vi "rio.vi"() -> ()   [LabVIEW 2012]
uses:
  <vilib>/rvi/interface/nirviOpenFPGA/nirviOpenFPGA.xnode
  <vilib>/rvi/interface/nirviMethod/nirviMethod.xnode
  <vilib>/rvi/interface/nirviReadWriteControl/nirviReadWriteControl.xnode
  <vilib>/addons/Fuzzy Logic/NI_Fuzzy_Logic_API.lvlib
  RIOGlobal.vi
  <vilib>/addons/Fuzzy Logic/TypeDefs/FL Interpolating polynomials.ctl
  <vilib>/addons/Fuzzy Logic/TypeDefs/FL Defuzzification.ctl
  <vilib>/addons/Fuzzy Logic/TypeDefs/FL Consequent Implication.ctl
  <vilib>/addons/Fuzzy Logic/TypeDefs/FL Modifier.ctl
  <vilib>/addons/Fuzzy Logic/TypeDefs/FL Consequent.ctl
  <vilib>/addons/Fuzzy Logic/TypeDefs/FL Antecedent Connective.ctl
  <vilib>/addons/Fuzzy Logic/TypeDefs/FL Antecedent.ctl
  <vilib>/addons/Fuzzy Logic/TypeDefs/FL Rule.ctl
  <vilib>/addons/Fuzzy Logic/TypeDefs/FL Membership Function Shape.ctl
  <vilib>/addons/Fuzzy Logic/TypeDefs/FL Membership Function.ctl
  <vilib>/addons/Fuzzy Logic/TypeDefs/FL Variable.ctl
  <vilib>/addons/Fuzzy Logic/TypeDefs/FL System.ctl
  <vilib>/FPGAPlugInAG/Dynamic/niLvFpga_Reset_Dynamic.vi
  <vilib>/rvi/interface/Simulation/niFpgaSimulationCallBeginRW.vi
  <vilib>/rvi/errors/niLvFpgaAdjustHostInterfaceError.vi
  <vilib>/FPGAPlugInAG/Dynamic/niLvFpga_Run_Dynamic.vi
  <vilib>/Utility/error.llb/Error Cluster From Error Code.vi
  NiFpgaLv.dll
  <vilib>/FPGAPlugInAG/Dynamic/niLvFpga_ReadFifo_Dynamic.vi
  <vilib>/rvi/errors/niLvFpgaMergeErrorWithErrorCode.vi
  logcode/G_read.vi
  <vilib>/FPGAPlugInAG/Dynamic/niLvFpga_StartFifo_Dynamic.vi
  <vilib>/addons/Fuzzy Logic/FL Fuzzy Controller (MISO).vi
  FPGA Bitfiles/autonomous_FPGATarget_autofpga8_egKHF51X6I0.lvbitx
  autocarnav4/soul/fpga/autofpga8.vi
  <vilib>/FPGAPlugInAG/cRIO-9114/niLvFpga_Open_cRIO-9114.vi
  <vilib>/rvi/interface/common/dynamic/niFpgaDynamicAddResources.vi
panel:
  out "get position":bool
  out "get heading":bool
  out "inbound?":bool
  in  "pos_error_bound gain":dbl=500.0
  out "LCC":dbl[](array[numeric]) format="%#_19f"
  out "tempheading":dbl
  in  "Buzz":bool=TRUE
  out "Steering_masual":dbl
  out "Steering_Des":dbl
  out "VS_Des":dbl
  out "Auto":bool
  out "Run":bool
  out "E - STOP":bool
  out "FPGA error out":errorcluster
  out "FPGA VI Reference Out":refnum<k20>
  out "bias":dbl
  in  "pos init manual":bool=TRUE
  out "hor.std.":dbl
  out "h_gps":dbl
  out "pos linit":bool
  out "dt":dbl
  out "ecef ref":dbl[](array[numeric])
  out "heading linit":bool
  out "time":i16
  out "output":T1
  in  "file write":bool
  out "refnum out":refnum<file>
  out "error out":errorcluster
  in  "position weight":dbl=0.1
  in  "heading weight":dbl=0.1
  out "rt":dbl
  out "steer_MDPS":dbl
  out "B Push percent x10":dbl
  in  "Slide":dbl(slide) scale=0.0..100.0
  in  "brake filter":dbl=1.0
  in  "Knob steer":dbl(knob)=122.29647676637626 scale=-550.0..550.0
  in  "knob steer":bool
  in  "auto brake":bool=TRUE
  in  "auto speed":bool=TRUE
  out "VS_TCU":dbl
  in  "auto steer":bool=TRUE
  out "Throttle Enable":bool=TRUE
  in  "VS_maual":dbl=33.0
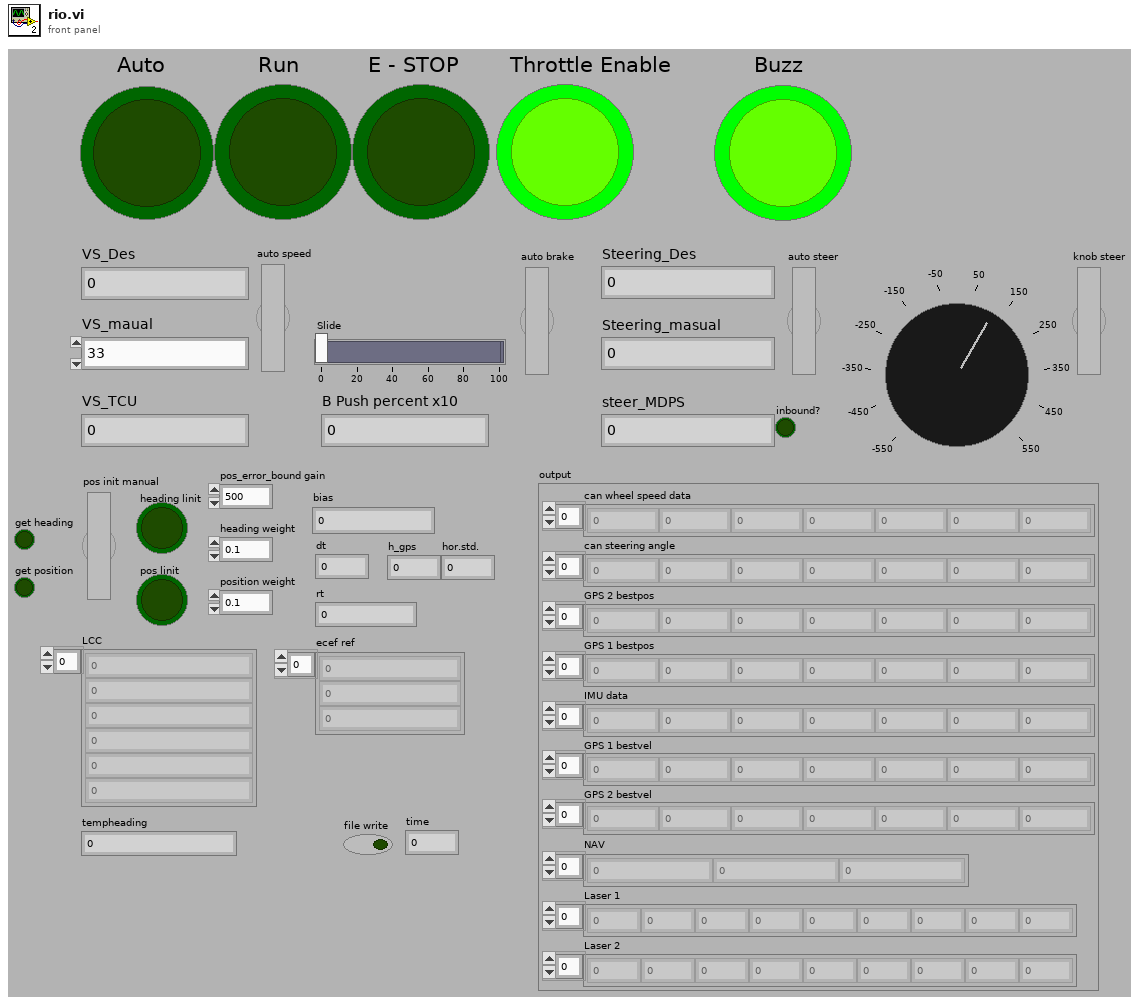
[diagram p1: front panel]
types:
  T1 = cluster{"can wheel speed data":u8[], "can steering angle":i32[], "GPS 2 bestpos":u8[], "GPS 1 bestpos":u8[], "IMU data":i16[], "GPS 1 bestvel":u8[], "GPS 2 bestvel":u8[], "NAV":dbl[], "Laser 1":u16[], "Laser 2":u16[]}
  T2 = typedef "NI_Fuzzy_Logic_API.lvlib/FL System.ctl" = cluster{"input variables":T3[], "output variables":T3[], "rules":T6[], "defuzzification method":T12, "description":string, "user MF interpolating polynomials":T13[]}
  T3 = typedef "NI_Fuzzy_Logic_API.lvlib/FL Variable.ctl" = cluster{"name":string, "range":dbl[], "MFs":T4[]}
  T4 = typedef "NI_Fuzzy_Logic_API.lvlib/FL Membership Function.ctl" = cluster{"name":string, "shape":T5, "points":dbl[], "color":u32, "user-defined shape index":i32}
  T5 = typedef "NI_Fuzzy_Logic_API.lvlib/FL Membership Function Shape.ctl" = u16
  T6 = typedef "NI_Fuzzy_Logic_API.lvlib/FL Rule.ctl" = cluster{"antecedents":T7[], "antecedent connective":T9, "consequents":T10[], "consequent implication":T11, "degree of support":dbl}
  T7 = typedef "NI_Fuzzy_Logic_API.lvlib/FL Antecedent.ctl" = cluster{"Var Index":i32, "MF Index":i32, "Cond":T8}
  T8 = typedef "NI_Fuzzy_Logic_API.lvlib/FL Modifier.ctl" = u16
  T9 = typedef "NI_Fuzzy_Logic_API.lvlib/FL Antecedent Connective.ctl" = u16
  T10 = typedef "NI_Fuzzy_Logic_API.lvlib/FL Consequent.ctl" = cluster{"Var Index":i32, "MF Index":i32, "Cond":T8}
  T11 = typedef "NI_Fuzzy_Logic_API.lvlib/FL Consequent Implication.ctl" = u16
  T12 = typedef "NI_Fuzzy_Logic_API.lvlib/FL Defuzzification.ctl" = u16
  T13 = typedef "NI_Fuzzy_Logic_API.lvlib/FL Interpolating polynomials.ctl" = cluster{"X":dbl[], "Y":dbl[], "Y(x) coeff":dbl[][], "X(y) coeff":dbl[][], "Area(y) coeff":dbl[][], "coa_x(y) coeff":dbl[][]}
  T14 = enum16{"open", "replace", "create", "open or create", "replace or create", "replace or create with confirmation"}
  T15 = cluster{"counter[ms]":u16, "rate x[rad/sec]":i16, "rate y[rad/sec]":i16, "rate z[rad/sec]":i16, "accel x[m/s^2]":i16, "accel y[m/s^2]":i16, "accel z[m/s^2]":i16}
  T16 = cluster{"counter[ms]":i16, "rate x[rad/sec]":i16, "rate y[rad/sec]":i16, "rate z[rad/sec]":i16, "accel x[m/s^2]":i16, "accel y[m/s^2]":i16, "accel z[m/s^2]":i16}
  T17 = cluster{"sol stat":u32, "vel type":u32, "latency":sgl, "age":sgl, "hor spd":dbl, "trk gnd":dbl, "vert spd":dbl, "reserved":sgl, "CRC":u32}
  T18 = cluster{"Sync_AA":u8, "Sync_44":u8, "Sync_12":u8, "Header Lgth":u8, "Message ID":u16, "Message Type":u8, "Port Address":u8, "Message Length":u16, "Sequence":u16, "Idle Time":u8, "Time Status":u8, "Week":u16, "ms":u32, "Receiver Status":u32, "Reserved":u16, "Receiver S/W Version":u16}
  T19 = cluster{"sol stat":u32, "pos type":u32, "lat":dbl, "lon":dbl, "hgt":dbl, "undulation":sgl, "dataum id":u32, "lat dev":sgl, "lon dev":sgl, "hgt dev":sgl, "stn id":u32, "diff_age":sgl, "sol_age":sgl, "#SVs":u8, "#solnSVs":u8, "#solnL1SVs":u8, "#solnMultiSVs":u8, "Reserved":u8, "ext sol stat":u8, "Reserved 2":u8, "sig mask":u8, "CRC":u32}
  T20 = cluster{"can wheel speed data":u8[], "can steering angle":i32[], "GPS 2 bestpos":u8[], "GPS 1 bestpos":u8[], "IMU data":i16[], "GPS 1 bestvel":u8[], "GPS 2 bestvel":u8[]}
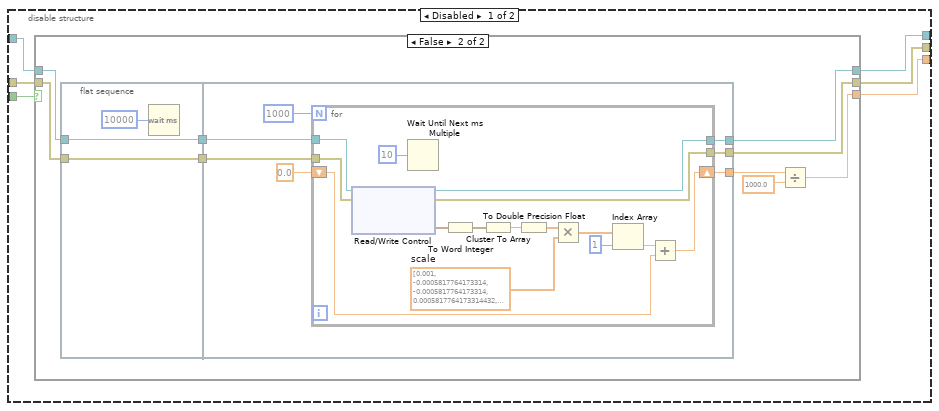
[diagram p2: hidden frame]
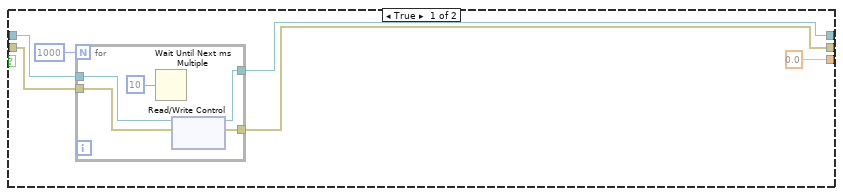
[diagram p3: hidden frame]
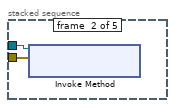
[diagram p4: hidden frame]
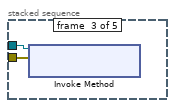
[diagram p5: hidden frame]
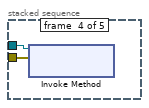
[diagram p6: hidden frame]
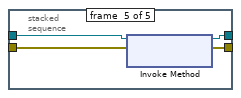
[diagram p7: hidden frame]
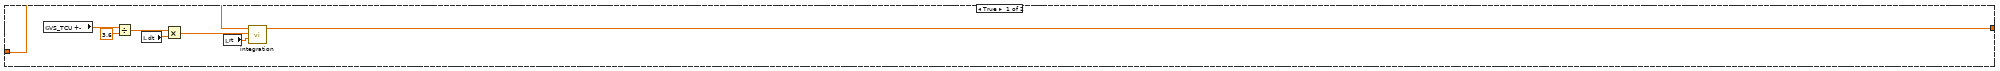
[diagram p12: hidden frame]
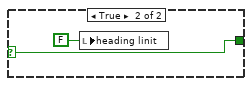
[diagram p13: hidden frame]
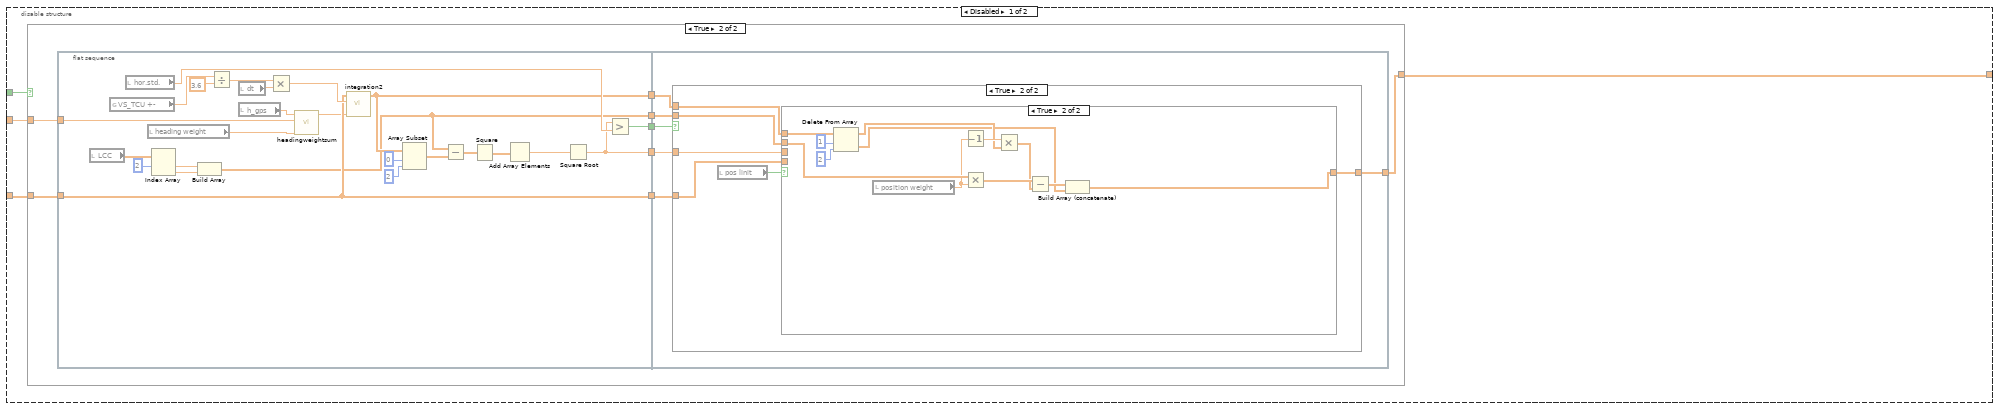
[diagram p14: hidden frame]
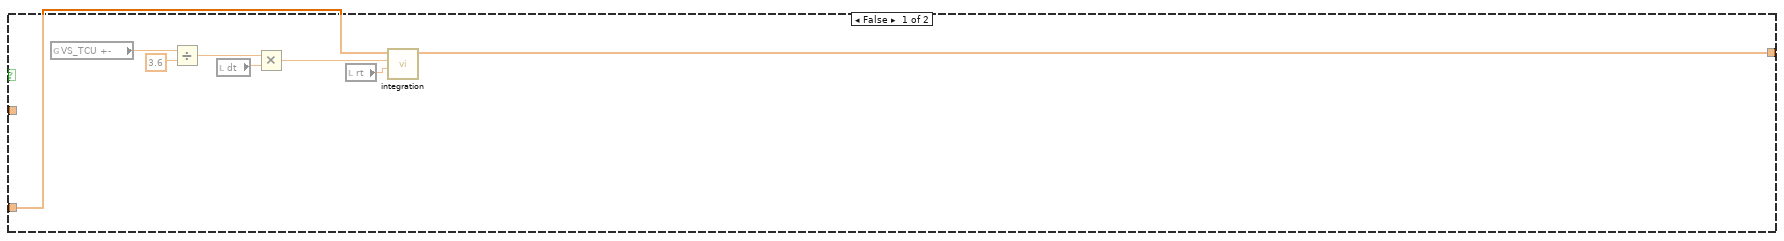
[diagram p15: hidden frame]
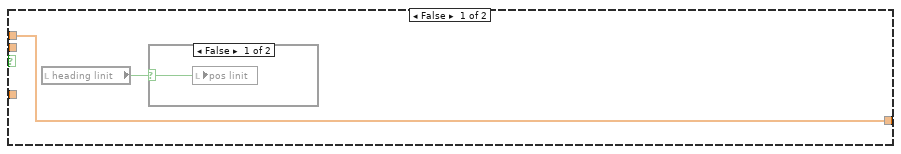
[diagram p16: hidden frame]
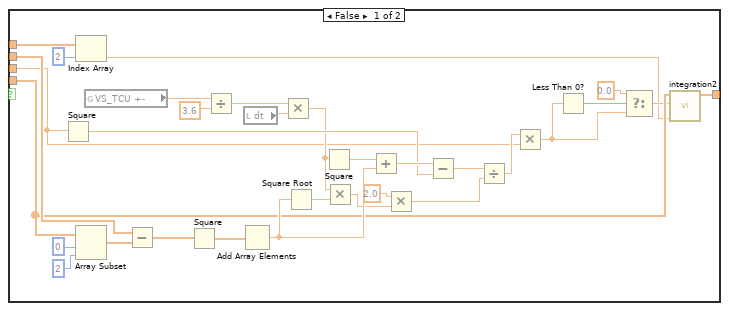
[diagram p18: hidden frame]
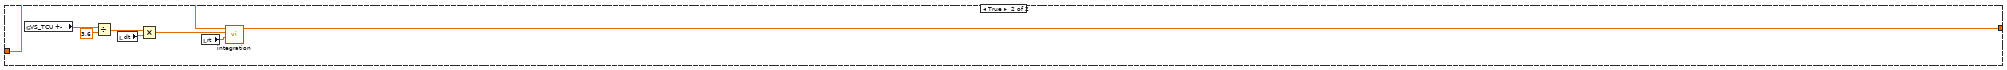
[diagram p19: hidden frame]
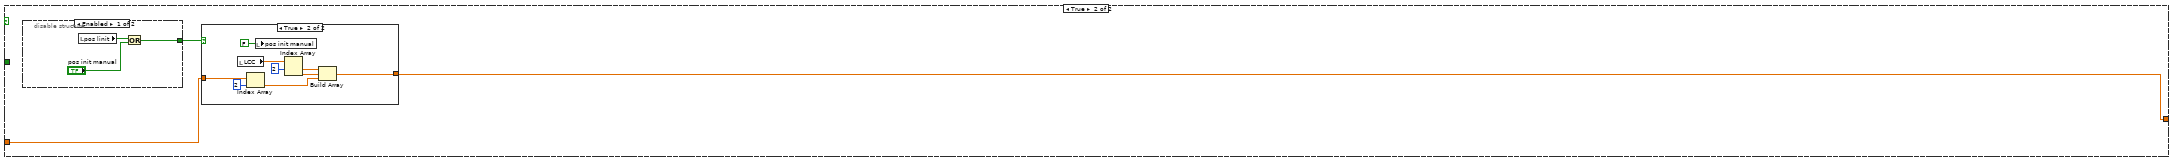
[diagram p20: hidden frame]
diagram:
  n1 = flat-sequence {
    tunnel: [T2 {"input variables"=[{"name"="Vdes-Vcar", "range"=[-100.0, 100.0, -150.0, 150.0], "MFs"=[{"name"="TF", "shape"=0, "points"=[-150.0, -10.0, -5.0], "color"=0, "user-defined shape index"=0}, {"name"="FR", "shape"=0, "points"=[-10.0, -5.0, 0.0], "color"=12369084, "user-defined shape index"=0}, {"name"="TR", "shape"=0, "points"=[-5.0, 0.0, 5.0], "color"=16711680, "user-defined shape index"=0}, {"name"="SR", "shape"=0, "points"=[0.0, 5.0, 10.0], "color"=6618880, "user-defined shape index"=0}, {"name"="TS", "shape"=0, "points"=[5.0, 10.0, 150.0], "color"=1985280, "user-defined shape index"=0}]}, {"name"="Vdes", "range"=[0.0, 10.0, -0.5, 100.0], "MFs"=[{"name"="ST", "shape"=0, "points"=[-0.5, 0.0, 0.5], "color"=16860, "user-defined shape index"=0}, {"name"="CR", "shape"=0, "points"=[0.0, 3.0, 6.0], "color"=16776704, "user-defined shape index"=0}, {"name"="DR", "shape"=0, "points"=[0.5, 10.0, 100.0], "color"=7171459, "user-defined shape index"=0}]}], "output variables"=[{"name"="BrakeAngle", "range"=[-5.0, 90.0, -5.0, 120.0], "MFs"=[{"name"="NB", "shape"=0, "points"=[-5.0, 0.0, 4.0], "color"=11121611, "user-defined shape index"=0}, {"name"="LB", "shape"=0, "points"=[0.0, 10.0, 20.0], "color"=11776947, "user-defined shape index"=0}, {"name"="MB", "shape"=0, "points"=[5.0, 35.0, 65.0], "color"=3381759, "user-defined shape index"=0}, {"name"="FB", "shape"=0, "points"=[20.0, 70.0, 120.0], "color"=32639, "user-defined shape index"=0}]}], "rules"=[{"antecedents"=[{"Var Index"=0, "MF Index"=0, "Cond"=0}, {"Var Index"=1, "MF Index"=0, "Cond"=0}], "antecedent connective"=0, "consequents"=[{"Var Index"=0, "MF Index"=3, "Cond"=0}], "consequent implication"=0, "degree of support"=1.0}, {"antecedents"=[{"Var Index"=0, "MF Index"=1, "Cond"=0}, {"Var Index"=1, "MF Index"=0, "Cond"=0}], "antecedent connective"=0, "consequents"=[{"Var Index"=0, "MF Index"=3, "Cond"=0}], "consequent implication"=0, "degree of support"=1.0}, {"antecedents"=[{"Var Index"=0, "MF Index"=2, "Cond"=0}, {"Var Index"=1, "MF Index"=0, "Cond"=0}], "antecedent connective"=0, "consequents"=[{"Var Index"=0, "MF Index"=2, "Cond"=0}], "consequent implication"=0, "degree of support"=1.0}, {"antecedents"=[{"Var Index"=0, "MF Index"=3, "Cond"=0}, {"Var Index"=1, "MF Index"=0, "Cond"=0}], "antecedent connective"=0, "consequents"=[{"Var Index"=0, "MF Index"=3, "Cond"=0}], "consequent implication"=0, "degree of support"=1.0}, {"antecedents"=[{"Var Index"=0, "MF Index"=4, "Cond"=0}, {"Var Index"=1, "MF Index"=0, "Cond"=0}], "antecedent connective"=0, "consequents"=[{"Var Index"=0, "MF Index"=3, "Cond"=0}], "consequent implication"=0, "degree of support"=1.0}, {"antecedents"=[{"Var Index"=0, "MF Index"=0, "Cond"=0}, {"Var Index"=1, "MF Index"=1, "Cond"=0}], "antecedent connective"=0, "consequents"=[{"Var Index"=0, "MF Index"=3, "Cond"=0}], "consequent implication"=0, "degree of support"=1.0}, {"antecedents"=[{"Var Index"=0, "MF Index"=1, "Cond"=0}, {"Var Index"=1, "MF Index"=1, "Cond"=0}], "antecedent connective"=0, "consequents"=[{"Var Index"=0, "MF Index"=2, "Cond"=0}], "consequent implication"=0, "degree of support"=1.0}, {"antecedents"=[{"Var Index"=0, "MF Index"=2, "Cond"=0}, {"Var Index"=1, "MF Index"=1, "Cond"=0}], "antecedent connective"=0, "consequents"=[{"Var Index"=0, "MF Index"=1, "Cond"=0}], "consequent implication"=0, "degree of support"=1.0}, {"antecedents"=[{"Var Index"=0, "MF Index"=3, "Cond"=0}, {"Var Index"=1, "MF Index"=1, "Cond"=0}], "antecedent connective"=0, "consequents"=[{"Var Index"=0, "MF Index"=0, "Cond"=0}], "consequent implication"=0, "degree of support"=1.0}, {"antecedents"=[{"Var Index"=0, "MF Index"=4, "Cond"=0}, {"Var Index"=1, "MF Index"=1, "Cond"=0}], "antecedent connective"=0, "consequents"=[{"Var Index"=0, "MF Index"=0, "Cond"=0}], "consequent implication"=0, "degree of support"=1.0}, {"antecedents"=[{"Var Index"=0, "MF Index"=0, "Cond"=0}, {"Var Index"=1, "MF Index"=2, "Cond"=0}], "antecedent connective"=0, "consequents"=[{"Var Index"=0, "MF Index"=3, "Cond"=0}], "consequent implication"=0, "degree of support"=1.0}, {"antecedents"=[{"Var Index"=0, "MF Index"=1, "Cond"=0}, {"Var Index"=1, "MF Index"=2, "Cond"=0}], "antecedent connective"=0, "consequents"=[{"Var Index"=0, "MF Index"=2, "Cond"=0}], "consequent implication"=0, "degree of support"=1.0}, {"antecedents"=[{"Var Index"=0, "MF Index"=2, "Cond"=0}, {"Var Index"=1, "MF Index"=2, "Cond"=0}], "antecedent connective"=0, "consequents"=[{"Var Index"=0, "MF Index"=0, "Cond"=0}], "consequent implication"=0, "degree of support"=1.0}, {"antecedents"=[{"Var Index"=0, "MF Index"=3, "Cond"=0}, {"Var Index"=1, "MF Index"=2, "Cond"=0}], "antecedent connective"=0, "consequents"=[{"Var Index"=0, "MF Index"=0, "Cond"=0}], "consequent implication"=0, "degree of support"=1.0}, {"antecedents"=[{"Var Index"=0, "MF Index"=4, "Cond"=0}, {"Var Index"=1, "MF Index"=2, "Cond"=0}], "antecedent connective"=0, "consequents"=[{"Var Index"=0, "MF Index"=0, "Cond"=0}], "consequent implication"=0, "degree of support"=1.0}], "defuzzification method"=0, "description"="", "user MF interpolating polynomials"=[]} ("fuzzy system out")] -> w1
    tunnel: w1 -> [w113]
    frame #0 {
      n2 = flat-sequence {
        frame #0 {
          w110 = TRUE ("auto steer")
          n3 = call "getecefdcmref.vi"("map"=2) -> ("XYZ"=→"ecef ref":dbl[])  [unwired: 10 in, 4 out]
          n4 = local write "Knob steer"(0.0 ("Knob steer")) -> ()
          n5 = local write "knob steer"(FALSE ("knob steer")) -> ()
          n6 = shared-variable "cRIO-9024\\sharedvari.lvlib\\parked"(FALSE ("parked")) -> ()  [unwired: 1 in, 1 out]
          n7 = local write "VS_maual"(32.0 ("VS_Desire")) -> ()
          n8 = global write "RIOGlobal.vi" "amp_ini"(2.5 ("amp_ini")) -> ()
          n9 = local write "Buzz"(w110) -> ()
          n10 = local write "auto steer"(w110) -> ()
          n11 = local write "auto speed"(w110) -> ()
          n12 = local write "auto brake"(w110) -> ()
          "heading linit" <- TRUE
          "pos linit" <- TRUE
        }
      }
      n13 = flat-sequence {
        frame #0 {
          n14 = xnode "Open FPGA VI Reference"() -> ("FPGA VI Reference Out"=w22:refnum<k20>, "error out"=w21:errorcluster)  [unwired: 2 in]
          n15 = xnode "Invoke Method"("FPGA VI Reference In"=w22, "error in"=w21) -> ("FPGA VI Reference Out"=w20:refnum<k20>, "error out"=w19:errorcluster)
          n16 = xnode "Read/Write Control"("FPGA VI Reference In"=w20, "error in"=w19, "read can"=TRUE, "16k"=FALSE) -> ("FPGA VI Reference Out"=w18:refnum<k20>, "error out"=w17:errorcluster)
          n17 = xnode "Invoke Method"("FPGA VI Reference In"=w18, "error in"=w17) -> ("FPGA VI Reference Out"=w15:refnum<k20>, "error out"=w14:errorcluster)  [unwired: 1 in]
          n18 = while {
            tunnel: w15 -> [w95]
            tunnel: w14 -> [w94]
            tunnel: [w93] -> w9
            tunnel: [w90] -> w10
            stop <- w91 stop-if-true
            n19 = xnode "Read/Write Control"("FPGA VI Reference In"=w95, "error in"=w94) -> ("FPGA VI Reference Out"=w90:refnum<k20>, "error out"=w93:errorcluster, "amp"=w92:fxp<+/-,16,5>)
            n20 = Not Equal To 0?(x=w92) -> (x != 0?=w91:bool)
          }
          n21 = stacked-sequence {
            tunnel: w10 -> [w79 w81 w83 w85 w89]
            tunnel: w9 -> [w78 w80 w82 w84 w88]
            tunnel: [_ _ _ _ w87] -> w7
            tunnel: [_ _ _ _ w86] -> w6
            frame #0 {
              n22 = xnode "Invoke Method"("FPGA VI Reference In"=w79, "error in"=w78) -> ()  [unwired: 2 out]
            }
            frame #1 {
              n23 = xnode "Invoke Method"("FPGA VI Reference In"=w81, "error in"=w80) -> ()  [unwired: 2 out]
            }
            frame #2 {
              n24 = xnode "Invoke Method"("FPGA VI Reference In"=w83, "error in"=w82) -> ()  [unwired: 2 out]
            }
            frame #3 {
              n25 = xnode "Invoke Method"("FPGA VI Reference In"=w85, "error in"=w84) -> ()  [unwired: 2 out]
            }
            frame #4 {
              n26 = xnode "Invoke Method"("FPGA VI Reference In"=w89, "error in"=w88) -> ("FPGA VI Reference Out"=w87:refnum<k20>, "error out"=w86:errorcluster)
            }
          }
          n27 = xnode "Read/Write Control"("FPGA VI Reference In"=w7, "error in"=w6) -> ("FPGA VI Reference Out"=w13:refnum<k20>, "error out"=w12:errorcluster, "IMU Connection error"=w11:bool)
          n28 = disable-structure shown="Enabled" {
            disable-tunnel: [w29 0.01 ("bias")] -> w5
            disable-tunnel: w13 -> [w28 w77]
            disable-tunnel: w12 -> [w27 w76]
            disable-tunnel: w11 -> [w26 _]
            disable-tunnel: [w25 w77] -> w4
            disable-tunnel: [w24 w76] -> w8
            frame Disabled {
              n29 = case shown="False" w26 {
                tunnel: [w35 w49] -> w25
                tunnel: [w34 w48] -> w24
                tunnel: [0.0 w41] -> w29
                tunnel: w28 -> [w33 w47]
                tunnel: w27 -> [w32 w46]
                frame True {
                  n30 = for {
                    N: 1000 -> [_]
                    tunnel: w33 -> [w40]
                    tunnel: [w39] -> w35
                    tunnel: w32 -> [w38]
                    tunnel: [w37] -> w34
                    n31 = Wait Until Next ms Multiple(millisecond multiple=u32 10) -> ()  [unwired: 1 out]
                    n32 = xnode "Read/Write Control"("FPGA VI Reference In"=w40, "error in"=w38) -> ("FPGA VI Reference Out"=w39:refnum<k20>, "error out"=w37:errorcluster)  [unwired: 1 out]
                  }
                }
                frame False {
                  n33 = flat-sequence {
                    tunnel: w46 -> [w51]
                    tunnel: w47 -> [w52]
                    tunnel: [w52] -> w45
                    tunnel: [w51] -> w44
                    tunnel: [w59] -> w49
                    tunnel: [w58] -> w48
                    tunnel: [w57] -> w42
                    tunnel: w45 -> [w56]
                    tunnel: w44 -> [w55]
                    frame #0 {
                      n34 = Wait (ms)(milliseconds to wait=u32 10000) -> ()  [unwired: 1 out]
                    }
                    frame #1 {
                      n35 = for {
                        N: 1000 -> [_]
                        tunnel: w56 -> [w74]
                        tunnel: [w73] -> w59
                        tunnel: w55 -> [w72]
                        tunnel: [w71] -> w58
                        shift-right: [w62] -> w57
                        shift-left: 0.0 -> [w61]
                        w66 = dbl[] [0.001, -0.0005817764173314, -0.0005817764173314, 0.0005817764173314432, -0.0032653, -0.0032653, 0.0032653]  # scale
                        n36 = xnode "Read/Write Control"("FPGA VI Reference In"=w74, "error in"=w72) -> ("FPGA VI Reference Out"=w73:refnum<k20>, "error out"=w71:errorcluster, "DATA IMU 1"=w68:T15)  [unwired: 1 out]
                        n37 = Wait Until Next ms Multiple(millisecond multiple=u32 10) -> ()  [unwired: 1 out]
                        n38 = To Word Integer(number=w68) -> (16bit integer=w70:T16)
                        n39 = Cluster To Array(cluster=w70) -> (array=w69:i16[])
                        n40 = To Double Precision Float(number=w69) -> (double precision float=w67:dbl[])
                        n41 = Multiply(x=w67, y=w66) -> (x*y=w65:dbl[])
                        n42 = Index Array(array=w65, index=1) -> (element=w63:dbl)
                        n43 = Add(x=w63, y=w61) -> (x+y=w62:dbl)
                      }
                    }
                  }
                  n44 = Divide(x=w42, y=1000.0) -> (x/y=w41:dbl)
                }
              }
            }
            frame Enabled {
            }
          }
          "bias" <- w5
          "FPGA VI Reference Out" <- w4
          "FPGA error out" <- w8
        }
      }
      n45 = case shown="True" "file write" {
        frame False {
        }
        frame True {
          n46 = Open/Create/Replace File(file path (use dialog)=path "c:/datasave", operation (0:open)=T14."replace or create", access (0:read/write)=enum16{"read/write", "read-only", "write-only"}."write-only") -> (refnum out=→"refnum out":refnum<file>, cancelled=w99:bool, error out=→"error out":errorcluster)  [unwired: 3 in]
          n47 = Not(x=w99) -> (.not. x?=w98:bool)
          n48 = local write "file write"(w98) -> ()
        }
      }
    }
    frame #1 {
      n49 = disable-structure shown="Enabled" {
        frame Enabled {
          n50 = while {
            stop <- FALSE stop-if-true
            n51 = local read "FPGA VI Reference Out"() -> (w601:refnum<k20>)
            n52 = xnode "Read/Write Control"("FPGA VI Reference In"=w601) -> ("FPGA VI Reference Out"=w604:refnum<k20>, "error out"=w605:errorcluster, "Connection error GPS 1"=w603:bool)  [unwired: 1 in]
            n53 = case shown="False" w603 {
              tunnel: w604 -> [w609 w668]
              tunnel: w605 -> [w608 w667]
              frame False {
                n54 = flat-sequence {
                  tunnel: w609 -> [w613]
                  tunnel: w608 -> [w612]
                  tunnel: [w611] -> w607
                  tunnel: [w610] -> w606
                  tunnel: w607 -> [w633]
                  tunnel: w606 -> [w632]
                  frame #0 {
                    n55 = while {
                      tunnel: w613 -> [w623]
                      tunnel: w612 -> [w622]
                      tunnel: [w615] -> w611
                      tunnel: [w614] -> w610
                      stop <- w616 stop-if-true
                      w621 = u32 1 ("Number of Elements")
                      n56 = xnode "Invoke Method"("FPGA VI Reference In"=w623, "error in"=w622, "Number of Elements"=w621, "Timeout (ms)"=w621) -> ("FPGA VI Reference Out"=w615:refnum<k20>, "error out"=w614:errorcluster, "Data"=w619:u8[])  [unwired: 1 out]
                      n57 = Index Array(array=w619, index=0) -> (element=w617:u8)
                      n58 = Equal?(x=w617, y=u8 170) -> (x = y?=w616:bool)
                    }
                  }
                  frame #1 {
                    w631 = u32 3 ("Number of Elements")
                    n59 = xnode "Invoke Method"("FPGA VI Reference In"=w633, "error in"=w632, "Number of Elements"=w631, "Timeout (ms)"=w631) -> ("FPGA VI Reference Out"=w626:refnum<k20>, "error out"=w625:errorcluster, "Data"=w629:u8[], "Elements Remaining"=w624:u32)
                    n60 = Equal?(x=w629, y=u8[] [68, 18, 28]) -> (x = y?=w628:bool[])
                    n61 = And Array Elements(Boolean array=w628) -> (logical AND=w627:bool)
                    n62 = case shown="True" w627 {
                      tunnel: w626 -> [w637 w643]
                      tunnel: w625 -> [w636 w642]
                      tunnel: w624 -> [w635 _]
                      frame False {
                        n63 = xnode "Invoke Method"("FPGA VI Reference In"=w637, "error in"=w636, "Number of Elements"=w635, "Timeout (ms)"=1) -> ()  [unwired: 4 out]
                      }
                      frame True {
                        w640 = u32 8 ("Number of Elements")
                        n64 = xnode "Invoke Method"("FPGA VI Reference In"=w643, "error in"=w642, "Number of Elements"=w640, "Timeout (ms)"=w640) -> ("FPGA VI Reference Out"=w656:refnum<k20>, "error out"=w657:errorcluster, "Data"=w659:u8[])  [unwired: 1 out]
                        n65 = Index Array(array=w659, index #1=1 ("index"), index #2=0 ("index"), index #3=5 ("index"), index #4=4 ("index")) -> (element #1=w646:u8, element #2=w647:u8, element #3=w651:u8, element #4=w652:u8)
                        n66 = Join Numbers(hi=w646, lo=w647) -> ((hi.lo)=w648:u16)
                        n67 = Join Numbers(hi=w651, lo=w652) -> ((hi.lo)=w653:u16)
                        n68 = Add(x=w653, y=u16 20) -> (x+y=w655:u16)
                        n69 = xnode "Invoke Method"("FPGA VI Reference In"=w656, "error in"=w657, "Number of Elements"=w655, "Timeout (ms)"=10) -> ("Data"=w639:u8[])  [unwired: 3 out]
                        n70 = Empty Array?(array=w639) -> (empty?=w638:bool)
                        n71 = Build Array (concatenate)(u8[] [170, 68, 18, 28], w659, w639) -> (w660:u8[])
                        n72 = case shown="False" w638 {
                          tunnel: w660 -> [w662 _]
                          tunnel: w648 -> [w661 _]
                          frame False {
                            n73 = case shown="99" w661 {
                              tunnel: w662 -> [_ w663 w664]
                              frame 0, Default {
                              }
                              frame 42 {
                                n74 = global write "G_read.vi" "GPS 1 bestpos"(w663) -> ()
                              }
                              frame 99 {
                                n75 = global write "G_read.vi" "GPS 1 bestvel"(w664) -> ()
                              }
                            }
                          }
                          frame True {
                          }
                        }
                      }
                    }
                  }
                }
              }
              frame True {
                n76 = xnode "Invoke Method"("FPGA VI Reference In"=w668, "error in"=w667, "Number of Elements"=u32 1, "Timeout (ms)"=5) -> ("FPGA VI Reference Out"=w670:refnum<k20>, "error out"=w671:errorcluster, "Elements Remaining"=w672:u32)  [unwired: 1 out]
                n77 = xnode "Invoke Method"("FPGA VI Reference In"=w670, "error in"=w671, "Number of Elements"=w672, "Timeout (ms)"=5) -> ()  [unwired: 4 out]
              }
            }
          }
          n78 = while {
            shift-right: [w120] -> _
            shift-left: dbl[] [0.0, 0.0, 0.0] ("pos") -> [w121]
            shift-right: [w118] -> _
            shift-left: i16 0 ("time") -> [w119]
            stop <- FALSE stop-if-true
            n79 = flat-sequence {
              tunnel: w119 -> [w124]
              tunnel: w121 -> [w125]
              tunnel: [w125] -> w117
              tunnel: [w124] -> w116
              tunnel: [w129] -> w120
              tunnel: [w127] -> w118
              tunnel: w117 -> [w130]
              tunnel: w116 -> [w128]
              frame #0 {
                n80 = Wait Until Next ms Multiple(millisecond multiple=u32 2) -> ()  [unwired: 1 out]
              }
              frame #1 {
                n81 = local read "FPGA VI Reference Out"() -> (w126:refnum<k20>)
                n82 = xnode "Read/Write Control"("FPGA VI Reference In"=w126) -> ("FPGA VI Reference Out"=w133:refnum<k20>, "error out"=w131:errorcluster, "IMU Connection error"=w132:bool)  [unwired: 1 in]
                n83 = case shown="False" w132 {
                  tunnel: w133 -> [w138 _]
                  tunnel: w131 -> [w137 _]
                  tunnel: w130 -> [w140 w600]
                  tunnel: [w139 w600] -> w129
                  tunnel: w128 -> [w136 w599]
                  tunnel: [w135 w599] -> w127
                  frame False {
                    n84 = flat-sequence {
                      tunnel: w138 -> [w196]
                      tunnel: w137 -> [w195]
                      tunnel: w140 -> [w193]
                      tunnel: [w192] -> w139
                      frame #0 {
                        n85 = flat-sequence {
                          tunnel: w196 -> [w218]
                          tunnel: w195 -> [w217]
                          tunnel: [w210] -> w194
                          frame #0 {
                            w208 = dbl[] [0.001, -0.0005817764173314, -0.0005817764173314, 0.0005817764173314432, -0.0032653, -0.0032653, 0.0032653]  # scale
                            n86 = xnode "Read/Write Control"("FPGA VI Reference In"=w218, "error in"=w217) -> ("DATA IMU 1"=w215:T15)  [unwired: 2 out]
                            n87 = To Word Integer(number=w215) -> (16bit integer=w216:T16)
                            n88 = Cluster To Array(cluster=w216) -> (array=w209:i16[])
                            n89 = To Double Precision Float(number=w209) -> (double precision float=w207:dbl[])
                            n90 = Multiply(x=w207, y=w208) -> (x*y=w206:dbl[])
                            n91 = local read "bias"() -> (w201:dbl)
                            n92 = Index Array(array=w206, index #1=0 ("index")) -> (element #1=w198:dbl, element #2=w204:dbl)  [unwired: 1 in]
                            n93 = Subtract(x=w198, y=0.01) -> (x-y=w200:dbl)
                            n94 = feedback #1(w200) -> (w197:dbl)
                            n95 = feedback-in #1(w198) -> ()
                            n96 = Subtract(x=w204, y=w201) -> (x-y=w202:dbl)
                            n97 = Subtract(x=w198, y=w197) -> (x-y=w211:dbl)
                            n98 = Increment(x=w211) -> (x+1=w212:dbl)
                            n99 = Less Than 0?(x=w211) -> (x < 0?=w213:bool)
                            n100 = Select(t=w212, s=w213, f=w211) -> (s? t:f=w203:dbl)
                            "dt" <- w203
                            n101 = Multiply(x=w203, y=w202) -> (x*y=→"rt":dbl)
                            n102 = Not Equal To 0?(x=w203) -> (x != 0?=w210:bool)
                          }
                        }
                        n103 = case shown="True" w194 {
                          tunnel: w193 -> [w219 w224]
                          tunnel: [w219 w221] -> w192
                          frame False {
                          }
                          frame True {
                            n104 = flat-sequence {
                              tunnel: w224 -> [w279]
                              tunnel: [w278] -> w222
                              tunnel: [w262] -> w223
                              frame #0 {
                                n105 = flat-sequence {
                                tunnel: [w303] -> w274
                                tunnel: [w302] -> w262
                                tunnel: [w285] -> w263
                                frame #0 {
                                n106 = local read "ecef ref"() -> (w301:dbl[])
                                n107 = global read "G_read.vi" "GPS 1 bestpos"() -> (w304:u8[])
                                n108 = global read "G_read.vi" "GPS 1 bestvel"() -> (w299:u8[])
                                n109 = call "gps_decode_bestvel.vi"("gps_data"=w299) -> ("checksum"=w284:bool, "vel"=w298:dbl[], "bestvel"=w295:T17, "log Header"=w292:T18)  [unwired: 7 in]
                                n110 = call "gps_decode.vi"("ecef ref"=w301, "gps_data"=w304) -> ("checksum"=w286:bool, "LCC"=w303:dbl[], "bestpos"=w302:T19)  [unwired: 6 in, 1 out]
                                "LCC" <- w303
                                n111 = Unbundle By Name(w295) -> ("sol stat"=w283:u32, "vel type"=w294:u32)
                                n112 = Unbundle By Name(w292) -> ("ms"=w290:u32)
                                n113 = Index Array(array=w298, index=4) -> (element=w296:dbl)
                                n114 = Equal To 0?(x=w283) -> (x = 0?=w281:bool)
                                n115 = call "angleconv.vi"("deg"=w296) -> ("rad"=→"h_gps":dbl)  [unwired: 9 in, 1 out]
                                n116 = Not(x=w286) -> (.not. x?=w285:bool)
                                n117 = Greater Or Equal?(x=w294, y=u32 8) -> (x >= y?=w288:bool)
                                n118 = feedback #2(u32 0 ("ms")) -> (w291:u32)
                                n119 = feedback-in #2(w290) -> ()
                                n120 = Not Equal?(x=w290, y=w291) -> (x != y?=w282:bool)
                                n121 = Compound Arithmetic op=AND(w282, w281, w288, w284) -> (→"get heading":bool)
                                }
                                }
                                n122 = global read "RIOGlobal.vi" "VS_TCU"() -> (w273:dbl)
                                n123 = Absolute Value(x=w273) -> (abs(x)=w272:dbl)
                                n124 = Equal To 0?(x=w272) -> (x = 0?=w280:bool)
                                n125 = Unbundle By Name(w262) -> ("sol stat"=w261:u32)
                                n126 = Index Array(array=w274, index #1=0 ("index")) -> (element #1=w271:dbl, element #2=w268:dbl)  [unwired: 1 in]
                                n127 = Equal To 0?(x=w271) -> (x = 0?=w270:bool)
                                n128 = feedback-in #3(w271) -> ()
                                n129 = feedback #3(0.0 ("Real Matrix Element")) -> (w275:dbl)
                                n130 = Less?(x=w268, y=16.0) -> (x < y?=w266:bool)
                                n131 = Equal?(x=w271, y=w275) -> (x = y?=w269:bool)
                                n132 = Not Equal To 0?(x=w261) -> (x != 0?=w260:bool)
                                n133 = Compound Arithmetic op=OR(w260, w269, w270, w266, w263) -> (w264:bool)
                                n134 = Not(x=w264) -> (.not. x?=→"get position":bool)
                                n135 = case shown="False" w280 {
                                tunnel: w279 -> [w307 w584]
                                tunnel: [w306 w583] -> w278
                                tunnel: w264 -> [w305 _]
                                frame False {
                                n136 = global read "RIOGlobal.vi" "VS_TCU +-"() -> (w311:dbl)
                                n137 = Absolute Value(x=w311) -> (abs(x)=w310:dbl)
                                n138 = Less?(x=w310, y=15.0) -> (x < y?=w308:bool)
                                n139 = case shown="False" w308 {
                                tunnel: w307 -> [w314 w577]
                                tunnel: [w312 w574] -> w306
                                tunnel: w305 -> [w313 _]
                                frame False {
                                n140 = case shown="False" w313 {
                                tunnel: w314 -> [w318 w325]
                                tunnel: [w317 w326] -> w312
                                frame True {
                                n141 = global read "RIOGlobal.vi" "VS_TCU +-"() -> (w322:dbl)
                                n142 = Divide(x=w322, y=3.6) -> (x/y=w320:dbl)
                                n143 = local read "dt"() -> (w319:dbl)
                                n144 = Multiply(x=w320, y=w319) -> (x*y=w316:dbl)
                                n145 = local read "rt"() -> (w315:dbl)
                                n146 = call "integration.vi"("rt"=w315, "dist"=w316, "pos(i-1)"=w318) -> ("pos(i)"=w317:dbl[])  [unwired: 8 in]
                                }
                                frame False {
                                n147 = flat-sequence {
                                tunnel: [w363] -> w327
                                tunnel: w325 -> [w335]
                                tunnel: [w352] -> w324
                                tunnel: [w335] -> w323
                                frame #0 {
                                w367 = 0.035  # 0.09
                                n148 = local read "LCC"() -> (w353:dbl[])
                                n149 = local read "LCC"() -> (w336:dbl[])
                                n150 = Array Subset(array=w335, index=0, length=2) -> (w344:dbl[])
                                n151 = Index Array(array=w335, index=2) -> (element=w355:dbl)
                                n152 = local read "get heading"() -> (w329:bool)
                                n153 = global read "RIOGlobal.vi" "VS_TCU +-"() -> (w331:dbl)
                                n154 = local read "rt"() -> (w364:dbl)
                                n155 = Index Array(array=w353, index #1=5 ("index")) -> (element #1=w361:dbl, element #2=w360:dbl)  [unwired: 1 in]
                                n156 = Array Subset(array=w336, index=2, length=2) -> (w343:dbl[])
                                n157 = call "headingoperater.vi"("h1"=w364, "h2"=w355) -> ("h2+h1"=w352:dbl)  [unwired: 8 in, 1 out]
                                n158 = local read "h_gps"() -> (w354:dbl)
                                n159 = Subtract(x=w343, y=w344) -> (x-y=w345:dbl[])
                                n160 = Square(x=w361) -> (x^2=w358:dbl)
                                n161 = Square(x=w360) -> (x^2=w359:dbl)
                                n162 = Absolute Value(x=w331) -> (abs(x)=w330:dbl)
                                n163 = Add(x=w358, y=w359) -> (x+y=w357:dbl)
                                n164 = call "headingoperater.vi"("h1"=w352, "h2"=w354) -> ("h2-h1"=w365:dbl)  [unwired: 8 in, 1 out]
                                n165 = Square(x=w345) -> (x^2=w346:dbl[])
                                n166 = Divide(x=w330, y=3.6) -> (x/y=w348:dbl)
                                n167 = Add Array Elements(numeric array=w346) -> (sum=w338:dbl)
                                n168 = Square Root(x=w357) -> (sqrt(x)=→"hor.std.":dbl)
                                n169 = local read "dt"() -> (w347:dbl)
                                n170 = Absolute Value(x=w365) -> (abs(x)=w366:dbl)
                                n171 = Multiply(x=w348, y=w347) -> (x*y=w350:dbl)
                                n172 = Less?(x=w366, y=w367) -> (x < y?=w333:bool)
                                n173 = Multiply(x=w350, y="pos_error_bound gain") -> (x*y=w351:dbl)
                                n174 = Square Root(x=w338) -> (sqrt(x)=w337:dbl)
                                n175 = Compound Arithmetic op=AND(w333, w329, w329) -> (w332:bool)
                                n176 = Less Or Equal?(x=w337, y=w351) -> (x <= y?=→"inbound?":bool)
                                n177 = case shown="False" w332 {
                                selector: w332 -> [_ w371]
                                tunnel: [w369 w371] -> w363
                                frame False {
                                n178 = local read "heading linit"() -> (w369:bool)
                                }
                                frame True {
                                n179 = local write "heading linit"(FALSE ("heading linit")) -> ()
                                }
                                }
                                }
                                }
                                n180 = disable-structure shown="Enabled" {
                                disable-tunnel: w327 -> [w375 w475]
                                disable-tunnel: [w374 w478] -> w326
                                disable-tunnel: w323 -> [w373 w477]
                                disable-tunnel: w324 -> [w372 w476]
                                frame Disabled {
                                n181 = case shown="True" w375 {
                                tunnel: [w377 w391] -> w374
                                tunnel: w373 -> [w376 w389]
                                tunnel: w372 -> [_ w384]
                                frame False {
                                n182 = global read "RIOGlobal.vi" "VS_TCU +-"() -> (w378:dbl)
                                n183 = Divide(x=w378, y=3.6) -> (x/y=w380:dbl)
                                n184 = local read "dt"() -> (w381:dbl)
                                n185 = Multiply(x=w380, y=w381) -> (x*y=w382:dbl)
                                n186 = local read "rt"() -> (w383:dbl)
                                n187 = call "integration.vi"("rt"=w383, "dist"=w382, "pos(i-1)"=w376) -> ("pos(i)"=w377:dbl[])  [unwired: 8 in]
                                }
                                frame True {
                                n188 = flat-sequence {
                                tunnel: [w396] -> w390
                                tunnel: w389 -> [w402]
                                tunnel: [w404] -> w388
                                tunnel: [w403] -> w387
                                tunnel: [w402] -> w386
                                tunnel: [w401] -> w385
                                tunnel: w384 -> [w394]
                                tunnel: [w422] -> w391
                                tunnel: w390 -> [w421]
                                tunnel: w388 -> [w420]
                                tunnel: w387 -> [w419]
                                tunnel: w386 -> [w418]
                                tunnel: w385 -> [w417]
                                frame #0 {
                                n189 = local read "LCC"() -> (w397:dbl[])
                                n190 = global read "RIOGlobal.vi" "VS_TCU +-"() -> (w416:dbl)
                                n191 = local read "hor.std."() -> (w405:dbl)
                                n192 = local read "heading weight"() -> (w392:dbl)
                                n193 = Index Array(array=w397, index #1=2 ("index")) -> (element #1=w399:dbl, element #2=w398:dbl)  [unwired: 1 in]
                                n194 = Build Array(w399, w398) -> (w396:dbl[])
                                n195 = Divide(x=w416, y=3.6) -> (x/y=w414:dbl)
                                n196 = local read "dt"() -> (w415:dbl)
                                n197 = local read "h_gps"() -> (w395:dbl)
                                n198 = Multiply(x=w414, y=w415) -> (x*y=w412:dbl)
                                n199 = call "headingweightsum.vi"("a"=w392, "h1"=w394, "h2"=w395) -> ("a*h2+(1-a)*h1"=w393:dbl)  [unwired: 8 in]
                                n200 = call "integration2.vi"("heading"=w393, "dist"=w412, "pos(i-1)"=w402) -> ("pos(i)"=w403:dbl[])  [unwired: 8 in]
                                n201 = Array Subset(array=w403, index=0, length=2) -> (w409:dbl[])
                                n202 = Subtract(x=w396, y=w409) -> (x-y=w408:dbl[])
                                n203 = Square(x=w408) -> (x^2=w407:dbl[])
                                n204 = Add Array Elements(numeric array=w407) -> (sum=w406:dbl)
                                n205 = Square Root(x=w406) -> (sqrt(x)=w401:dbl)
                                n206 = Greater?(x=w401, y=w405) -> (0:w404:bool)
                                }
                                frame #1 {
                                n207 = case shown="True" w420 {
                                tunnel: [w423 w429] -> w422
                                tunnel: w421 -> [_ w430]
                                tunnel: w419 -> [w423 w428]
                                tunnel: w418 -> [_ w427]
                                tunnel: w417 -> [_ w426]
                                frame False {
                                n208 = local read "heading linit"() -> (w424:bool)
                                n209 = case shown="False" w424 {
                                selector: w424 -> [w425 _]
                                frame False {
                                n210 = local write "pos linit"(w425) -> ()
                                }
                                frame True {
                                }
                                }
                                }
                                frame True {
                                n211 = local read "pos linit"() -> (w431:bool)
                                n212 = case shown="True" w431 {
                                tunnel: w430 -> [w458 w474]
                                tunnel: [w432 w469] -> w429
                                tunnel: w428 -> [w435 w468]
                                tunnel: w427 -> [w437 _]
                                tunnel: w426 -> [w442 _]
                                frame False {
                                n213 = Square(x=w442) -> (x^2=w450:dbl)
                                n214 = Index Array(array=w435, index=2) -> (element=w433:dbl)
                                n215 = Array Subset(array=w437, index=0, length=2) -> (w462:dbl[])
                                n216 = global read "RIOGlobal.vi" "VS_TCU +-"() -> (w454:dbl)
                                n217 = Subtract(x=w458, y=w462) -> (x-y=w461:dbl[])
                                n218 = Square(x=w461) -> (x^2=w460:dbl[])
                                n219 = Divide(x=w454, y=3.6) -> (x/y=w456:dbl)
                                n220 = Add Array Elements(numeric array=w460) -> (sum=w452:dbl)
                                n221 = local read "dt"() -> (w455:dbl)
                                n222 = Multiply(x=w456, y=w455) -> (x*y=w448:dbl)
                                n223 = Square Root(x=w452) -> (sqrt(x)=w449:dbl)
                                n224 = Square(x=w448) -> (x^2=w453:dbl)
                                n225 = Multiply(x=w448, y=w449) -> (x*y=w447:dbl)
                                n226 = Add(x=w453, y=w452) -> (x+y=w451:dbl)
                                n227 = Multiply(x=2.0, y=w447) -> (x*y=w444:dbl)
                                n228 = Subtract(x=w451, y=w450) -> (x-y=w445:dbl)
                                n229 = Divide(x=w445, y=w444) -> (x/y=w443:dbl)
                                n230 = Multiply(x=w443, y=w442) -> (x*y=w438:dbl)
                                n231 = Less Than 0?(x=w438) -> (x < 0?=w440:bool)
                                n232 = Select(t=0.0, s=w440, f=w438) -> (s? t:f=w436:dbl)
                                n233 = call "integration2.vi"("heading"=w433, "dist"=w436, "pos(i-1)"=w437) -> ("pos(i)"=w432:dbl[])  [unwired: 8 in]
                                }
                                frame True {
                                n234 = Delete From Array(array=w468, length=1, index=2) -> (deleted portion=w464:dbl[], array with subset deleted=w465:dbl[])
                                n235 = local read "position weight"() -> (w463:dbl)
                                n236 = Decrement(x=w463) -> (x-1=w473:dbl)
                                n237 = Multiply(x=w474, y=w463) -> (x*y=w472:dbl[])
                                n238 = Multiply(x=w473, y=w465) -> (x*y=w471:dbl[])
                                n239 = Subtract(x=w472, y=w471) -> (x-y=w470:dbl[])
                                n240 = Build Array (concatenate)(w470, w464) -> (w469:dbl[])
                                }
                                }
                                }
                                }
                                }
                                }
                                }
                                }
                                }
                                frame Enabled {
                                n241 = flat-sequence {
                                tunnel: w477 -> [w486]
                                tunnel: w476 -> [w487]
                                tunnel: [w484] -> w478
                                tunnel: w475 -> [w480]
                                frame #0 {
                                n242 = flat-sequence {
                                tunnel: w487 -> [w490]
                                tunnel: w486 -> [w488]
                                tunnel: [w492] -> w485
                                tunnel: [w489] -> w481
                                tunnel: w480 -> [w491]
                                tunnel: [w488] -> w479
                                tunnel: w485 -> [w511]
                                tunnel: [w512] -> w483
                                tunnel: [w511] -> w482
                                tunnel: w481 -> [w510]
                                tunnel: w479 -> [w504]
                                tunnel: [w531] -> w484
                                tunnel: w483 -> [w530]
                                tunnel: w482 -> [w529]
                                frame #0 {
                                n243 = case shown="True" w491 {
                                tunnel: w490 -> [w498 w501]
                                tunnel: [w498 w500] -> w489
                                frame False {
                                }
                                frame True {
                                n244 = local read "heading weight"() -> (w499:dbl)
                                n245 = local read "h_gps"() -> (w502:dbl)
                                n246 = call "headingweightsum.vi"("a"=w499, "h1"=w501, "h2"=w502) -> ("a*h2+(1-a)*h1"=w500:dbl)  [unwired: 8 in]
                                }
                                }
                                n247 = global read "RIOGlobal.vi" "VS_TCU +-"() -> (w493:dbl)
                                n248 = Divide(x=w493, y=3.6) -> (x/y=w495:dbl)
                                n249 = local read "dt"() -> (w494:dbl)
                                n250 = Multiply(x=w495, y=w494) -> (x*y=w497:dbl)
                                n251 = call "integration2.vi"("heading"=w489, "dist"=w497, "pos(i-1)"=w488) -> ("pos(i)"=w492:dbl[])  [unwired: 8 in]
                                }
                                frame #1 {
                                n252 = local read "LCC"() -> (w506:dbl[])
                                n253 = Delete From Array(array=w511, length=1, index=2) -> (deleted portion=w526:dbl[], array with subset deleted=w525:dbl[])
                                n254 = local read "position weight"() -> (w527:dbl)
                                n255 = Index Array(array=w506, index #1=2 ("index")) -> (element #1=w508:dbl, element #2=w507:dbl)  [unwired: 1 in]
                                n256 = Build Array(w508, w507) -> (w505:dbl[])
                                n257 = Multiply(x=w505, y=w527) -> (x*y=w520:dbl[])
                                n258 = Decrement(x=w527) -> (x-1=w519:dbl)
                                n259 = Multiply(x=w519, y=w525) -> (x*y=w521:dbl[])
                                n260 = Subtract(x=w520, y=w521) -> (x-y=w522:dbl[])
                                n261 = Build Array (concatenate)(w522, w526) -> (w512:dbl[])
                                n262 = Subtract(x=w512, y=w504) -> (x-y=w518:dbl[])
                                n263 = Index Array(array=w518, index #1=1 ("index"), index #2=0 ("index")) -> (element #1=w516:dbl, element #2=w515:dbl)
                                n264 = Inverse Tangent (2 Input)(1:w515, 2:w516) -> (0:w514:dbl)
                                n265 = call "headingoperater.vi"("h1"=w510, "h2"=w514) -> ("h2-h1"=→"tempheading":dbl)  [unwired: 8 in, 1 out]
                                }
                                frame #2 {
                                n266 = local read "heading linit"() -> (w528:bool)
                                n267 = case shown="False" w528 {
                                tunnel: [w537 w573] -> w531
                                tunnel: w530 -> [w536 w573]
                                tunnel: w529 -> [w535 _]
                                frame False {
                                n268 = local read "inbound?"() -> (w532:bool)
                                n269 = local read "tempheading"() -> (w540:dbl)
                                n270 = Absolute Value(x=w540) -> (abs(x)=w539:dbl)
                                n271 = Less?(x=w539, y=0.17453292519943295) -> (x < y?=w533:bool)
                                n272 = And(x=w532, y=w533) -> (x .and. y?=w534:bool)
                                n273 = case shown="False" w534 {
                                tunnel: [w543 w571] -> w537
                                tunnel: w536 -> [_ w571]
                                tunnel: w535 -> [w542 _]
                                tunnel: w532 -> [w541 _]
                                frame False {
                                n274 = local read "hor.std."() -> (w548:dbl)
                                n275 = local read "tempheading"() -> (w550:dbl)
                                n276 = Less?(x=w548, y=16.0) -> (x < y?=w545:bool)
                                n277 = Absolute Value(x=w550) -> (abs(x)=w551:dbl)
                                n278 = Less?(x=w551, y=0.7853981633974483) -> (x < y?=w546:bool)
                                n279 = Compound Arithmetic op=AND(w545, w546, w541) -> (w544:bool)
                                n280 = case shown="True" w544 {
                                tunnel: [w552 w561] -> w543
                                tunnel: w542 -> [w552 w562]
                                frame False {
                                }
                                frame True {
                                n281 = local read "LCC"() -> (w557:dbl[])
                                n282 = Delete From Array(array=w562, length=1, index=2) -> (deleted portion=w570:dbl[], array with subset deleted=w569:dbl[])
                                n283 = local read "position weight"() -> (w560:dbl)
                                n284 = Index Array(array=w557, index #1=2 ("index")) -> (element #1=w555:dbl, element #2=w556:dbl)  [unwired: 1 in]
                                n285 = Build Array(w555, w556) -> (w553:dbl[])
                                n286 = Multiply(x=w560, y=0.2) -> (x*y=w558:dbl)
                                n287 = Multiply(x=w553, y=w558) -> (x*y=w564:dbl[])
                                n288 = Decrement(x=w558) -> (x-1=w563:dbl)
                                n289 = Multiply(x=w563, y=w569) -> (x*y=w565:dbl[])
                                n290 = Subtract(x=w564, y=w565) -> (x-y=w566:dbl[])
                                n291 = Build Array (concatenate)(w566, w570) -> (w561:dbl[])
                                }
                                }
                                }
                                frame True {
                                n292 = local read "heading linit"() -> (w572:bool)
                                n293 = local write "pos linit"(w572) -> ()
                                }
                                }
                                }
                                frame True {
                                }
                                }
                                }
                                }
                                }
                                }
                                }
                                }
                                }
                                }
                                }
                                frame True {
                                n294 = global read "RIOGlobal.vi" "VS_TCU +-"() -> (w581:dbl)
                                n295 = Divide(x=w581, y=3.6) -> (x/y=w579:dbl)
                                n296 = local read "dt"() -> (w578:dbl)
                                n297 = Multiply(x=w579, y=w578) -> (x*y=w576:dbl)
                                n298 = local read "rt"() -> (w575:dbl)
                                n299 = call "integration.vi"("rt"=w575, "dist"=w576, "pos(i-1)"=w577) -> ("pos(i)"=w574:dbl[])  [unwired: 8 in]
                                }
                                }
                                }
                                frame True {
                                n300 = disable-structure shown="Enabled" {
                                disable-tunnel: [w585 TRUE] -> w582
                                frame Enabled {
                                n301 = local read "pos linit"() -> (w587:bool)
                                n302 = Or(x=w587, y="pos init manual") -> (x .or. y?=w585:bool)
                                }
                                frame Disabled {
                                }
                                }
                                n303 = case shown="True" w582 {
                                tunnel: w584 -> [w589 w597]
                                tunnel: [w589 w592] -> w583
                                frame False {
                                }
                                frame True {
                                n304 = local read "LCC"() -> (w590:dbl[])
                                n305 = Index Array(array=w597, index=2) -> (element=w593:dbl)
                                n306 = local write "pos init manual"(FALSE ("Buzz 2")) -> ()
                                n307 = Index Array(array=w590, index #1=2 ("index")) -> (element #1=w595:dbl, element #2=w594:dbl)  [unwired: 1 in]
                                n308 = Build Array(w595, w594, w593) -> (w592:dbl[])
                                }
                                }
                                }
                                }
                              }
                            }
                            n309 = flat-sequence {
                              tunnel: w223 -> [w259]
                              tunnel: w222 -> [w225]
                              tunnel: [w230] -> w220
                              tunnel: [w225] -> w221
                              frame #0 {
                                n310 = global write "G_read.vi" "NAV"(w225) -> ()
                                n311 = local read "LCC"() -> (w229:dbl[])
                                n312 = local read "LCC"() -> (w227:dbl[])
                                n313 = Unbundle By Name(w259) -> ("#SVs"=w256:u8, "pos type"=w253:u32, "lat dev"=w251:sgl, "lon dev"=w250:sgl, "hgt dev"=w249:sgl, "lat"=w248:dbl, "lon"=w247:dbl, "hgt"=w246:dbl)
                                n314 = local read "ecef ref"() -> (w232:dbl[])
                                n315 = Index Array(array=w229, index=0) -> (element=w257:dbl)
                                n316 = Index Array(array=w227, index=4) -> (element=w226:dbl)
                                n317 = Index Array(array=w225, index #1=0 ("index")) -> (element #1=w241:dbl, element #2=w240:dbl, element #3=w234:dbl)  [unwired: 2 in]
                                n318 = global read "G_read.vi" "GPS 2 bestpos"() -> (w255:u8[])
                                n319 = Less Than 0?(x=w234) -> (x < 0?=w236:bool)
                                n320 = Add(x=w234, y=6.283185307179586) -> (x+y=w235:dbl)
                                n321 = Select(t=w235, s=w236, f=w234) -> (s? t:f=w233:dbl)
                                n322 = call "gps_decode.vi"("ecef ref"=w232, "gps_data"=w255) -> ("bestpos"=w254:T19)  [unwired: 6 in, 3 out]
                                n323 = Unbundle By Name(w254) -> ("diff_age"=w252:sgl, "lat"=w245:dbl, "lon"=w244:dbl, "hgt"=w243:dbl)
                                n324 = local read "h_gps"() -> (w231:dbl)
                                n325 = Build Array(w257, w256, w253, w252, w251, w250, w249, w248, w247, w246, w245, w244, w243, w241, w240, w226, 0.0 ("element"), 0.0 ("element"), w233, w231) -> (w230:dbl[])
                                n326 = global write "G_read.vi" "RIONAV"(w230) -> ()
                              }
                            }
                            n327 = shared-variable "cRIO-9024\\sharedvari.lvlib\\RIONAV"(w220) -> ()  [unwired: 1 in, 1 out]
                          }
                        }
                      }
                    }
                    n328 = local read "file write"() -> (w134:bool)
                    n329 = case shown="True" w134 {
                      tunnel: w138 -> [_ w144]
                      tunnel: w137 -> [_ w143]
                      tunnel: w136 -> [_ w142]
                      tunnel: [_ w141] -> w135
                      frame False {
                      }
                      frame True {
                        n330 = flat-sequence {
                          tunnel: w144 -> [w183]
                          tunnel: w143 -> [w182]
                          tunnel: [w157] -> w141
                          tunnel: w142 -> [w155]
                          frame #0 {
                            (unwired) T20 {"can wheel speed data"=[], "can steering angle"=[], "GPS 2 bestpos"=[], "GPS 1 bestpos"=[], "IMU data"=[], "GPS 1 bestvel"=[], "GPS 2 bestvel"=[]} ("output")
                            n331 = xnode "Read/Write Control"("FPGA VI Reference In"=w183, "error in"=w182) -> ("DATA IMU 1"=w151:T15, "SAS_angle_MDPS"=w152:i32, "WHEEL_FL"=w181:u8, "WHEEL_FRFL"=w180:u8, "WHEEL_FR"=w179:u8, "WHEEL_RL"=w178:u8, "WHEEL_RRRL"=w177:u8, "WHELL_RR"=w176:u8, "G_sel_disp"=w175:u8)  [unwired: 2 out]
                            n332 = To Long Integer(number=0) -> (32bit integer=w174:i32)
                            n333 = Build Array(u8 0 ("element"), w181, w180, w179, w178, w177, w176, w175) -> (w172:u8[])
                            n334 = To Word Integer(number=w151) -> (16bit integer=w184:T16)
                            n335 = Build Array(w174, w152) -> (w173:i32[])
                            n336 = global read "G_read.vi" "Laser 2"() -> (w148:u16[])
                            n337 = global read "G_read.vi" "Laser 1"() -> (w149:u16[])
                            n338 = global read "G_read.vi" "GPS 1 bestpos"() -> (w169:u8[])
                            n339 = global read "G_read.vi" "GPS 2 bestpos"() -> (w168:u8[])
                            n340 = global read "G_read.vi" "GPS 1 bestvel"() -> (w166:u8[])
                            n341 = global read "G_read.vi" "GPS 2 bestvel"() -> (w167:u8[])
                            n342 = Cluster To Array(cluster=w184) -> (array=w159:i16[])
                            n343 = global read "G_read.vi" "NAV"() -> (w145:dbl[])
                            n344 = Index Array(array=w159, index=0) -> (element=w156:i16)
                            n345 = Build Array (concatenate)(u8 0 ("unsigned 8bit integer"), w166) -> (w165:u8[])
                            n346 = Build Array (concatenate)(u8 0 ("unsigned 8bit integer"), w167) -> (w164:u8[])
                            n347 = Build Array (concatenate)(u8 0 ("unsigned 8bit integer"), w169) -> (w171:u8[])
                            n348 = Build Array (concatenate)(u8 0 ("unsigned 8bit integer"), w168) -> (w170:u8[])
                            n349 = Bundle By Name(cluster=T1 {"can wheel speed data"=[], "can steering angle"=[], "GPS 2 bestpos"=[], "GPS 1 bestpos"=[], "IMU data"=[], "GPS 1 bestvel"=[], "GPS 2 bestvel"=[], "NAV"=[], "Laser 1"=[], "Laser 2"=[]} ("output"), "IMU data"=w159, "can steering angle"=w173, "can wheel speed data"=w172, "GPS 1 bestpos"=w171, "GPS 2 bestpos"=w170, "GPS 1 bestvel"=w165, "GPS 2 bestvel"=w164, "Laser 1"=w149, "Laser 2"=w148, "NAV"=w145) -> (w147:T1)
                            "output" <- w147
                            n350 = Not Equal?(x=w155, y=w156) -> (x != y?=w150:bool)
                            n351 = case shown="True" w150 {
                              tunnel: w147 -> [_ w190]
                              tunnel: [w185 w188] -> w157
                              tunnel: w156 -> [_ w188]
                              tunnel: w155 -> [w185 w187]
                              frame False {
                              }
                              frame True {
                                n352 = Subtract(x=w188, y=w187) -> (x-y=→"time":i16)
                                n353 = local read "refnum out"() -> (w191:refnum<file>)
                                n354 = Write to Binary File(file (use dialog)=w191, data=w190) -> (error out=w189:errorcluster)  [unwired: 4 in, 2 out]
                                n355 = local write "error out"(w189) -> ()
                              }
                            }
                          }
                        }
                      }
                    }
                  }
                  frame True {
                  }
                }
              }
            }
          }
        }
        frame Disabled {
        }
      }
      n356 = disable-structure shown="Enabled" {
        disable-tunnel: w113 -> [w673]
        frame Enabled {
          n357 = while {
            stop <- FALSE stop-if-true
            n358 = flat-sequence {
              frame #0 {
                n359 = Wait Until Next ms Multiple(millisecond multiple=u32 5) -> ()  [unwired: 1 out]
              }
              frame #1 {
                n360 = local read "FPGA VI Reference Out"() -> (w676:refnum<k20>)
                n361 = call "datadecoder.vi"("FPGA VI Reference Out"=w676) -> ()  [unwired: 7 in]
              }
              frame #2 {
                n362 = global read "RIOGlobal.vi" "Auto"() -> (w682:bool)
                "Auto" <- w682
                n363 = global read "RIOGlobal.vi" "Run"() -> (w681:bool)
                "Run" <- w681
                n364 = global read "RIOGlobal.vi" "VS_TCU +-"() -> (→"VS_TCU":dbl)
                n365 = global read "RIOGlobal.vi" "SAS_angle_MDPS"() -> (→"steer_MDPS":dbl)
                n366 = global read "RIOGlobal.vi" "Throttle_Enable"() -> (→"Throttle Enable":bool)
                n367 = Not(x=w681) -> (.not. x?=w680:bool)
                n368 = And(x=w682, y=w680) -> (x .and. y?=→"E - STOP":bool)
              }
              frame #3 {
                n369 = local read "FPGA VI Reference Out"() -> (w684:refnum<k20>)
                n370 = call "dataencoder.vi"("Buzz"="Buzz", "auto steer"="auto steer", "FPGA VI Reference In"=w684) -> ()  [unwired: 9 in]
              }
            }
          }
          n371 = while {
            stop <- FALSE stop-if-true
            n372 = flat-sequence {
              frame #0 {
                n373 = global read "RIOGlobal.vi" "SAS_angle_MDPS"() -> (w825:dbl)
                n374 = shared-variable "cRIO-9024\\sharedvari.lvlib\\steer_input"() -> (w818:dbl)  [unwired: 1 in, 1 out]
                n375 = feedback #4(0.0 ("Double")) -> (w829:dbl)
                n376 = Not A Number/Path/Refnum?(number/path/refnum=w818) -> (NaN/Path/Refnum?=w817:bool)
                n377 = Select(t=w829, s=w817, f=w818) -> (s? t:f=w831:dbl)
                n378 = feedback-in #4(w831) -> ()
                n379 = Select(t="Knob steer", s="knob steer", f=w831) -> (s? t:f=w832:dbl)
                n380 = call "lpf3.vi"("filter_gain"=0.95 ("filter_R"), "In1"=w832) -> ("Out1"=w833:dbl)  [unwired: 9 in]
                n381 = In Range and Coerce(upper limit=510.0 ("max"), x=w833, lower limit=-510.0 ("min")) -> (coerced(x)=w828:dbl)  [unwired: 1 out]
                n382 = Subtract(x=w828, y=w825) -> (x-y=w819:dbl)
                n383 = In Range and Coerce(upper limit=100.0, x=w819, lower limit=-100.0) -> (coerced(x)=w824:dbl, In Range?=w822:bool)
                n384 = case shown="False" w822 {
                  tunnel: [w838 w839] -> w823
                  tunnel: w828 -> [_ w839]
                  tunnel: w824 -> [w836 _]
                  frame False {
                    n385 = global read "RIOGlobal.vi" "SAS_angle_MDPS"() -> (w837:dbl)
                    n386 = Multiply(x=w836, y=0.5) -> (x*y=w834:dbl)
                    n387 = Add(x=w837, y=w834) -> (x+y=w838:dbl)
                  }
                  frame True {
                  }
                }
                n388 = global write "RIOGlobal.vi" "MDPS_Control"(w823) -> ()
                "Steering_masual" <- "Knob steer"
              }
            }
            n389 = flat-sequence {
              frame #0 {
                n390 = case shown="True" "auto speed" {
                  tunnel: ["VS_maual" w863] -> w841
                  frame False {
                  }
                  frame True {
                    n391 = shared-variable "cRIO-9024\\sharedvari.lvlib\\vs_des"() -> (w871:dbl)  [unwired: 1 in, 1 out]
                    n392 = local read "auto steer"() -> (w862:bool)
                    n393 = global read "RIOGlobal.vi" "VS_saved"() -> (w869:dbl)
                    n394 = global read "RIOGlobal.vi" "SAS_angle_MDPS"() -> (w868:dbl)
                    n395 = shared-variable "cRIO-9024\\sharedvari.lvlib\\steer_input"() -> (w858:dbl)  [unwired: 1 in, 1 out]
                    "Steering_Des" <- w858
                    n396 = Not A Number/Path/Refnum?(number/path/refnum=w871) -> (NaN/Path/Refnum?=w870:bool)
                    n397 = Subtract(x=w868, y=w858) -> (x-y=w867:dbl)
                    n398 = Select(t=w869, s=w870, f=w871) -> (s? t:f=w859:dbl)
                    "VS_Des" <- w859
                    n399 = Absolute Value(x=w867) -> (abs(x)=w866:dbl)
                    n400 = Select(t=0.0, s=w862, f=w859) -> (s? t:f=w860:dbl)
                    n401 = Greater Or Equal?(x=w866, y=100.0 ("steering offset")) -> (x >= y?=w864:bool)
                    n402 = Select(t=w860, s=w864, f=w859) -> (s? t:f=w863:dbl)
                  }
                }
                n403 = global write "RIOGlobal.vi" "VS_saved"(w841) -> ()
                n404 = Sign(1:w841) -> (0:w842:dbl)
                n405 = case shown="-1" w842 {
                  tunnel: [w846 _ w853] -> w840
                  tunnel: w841 -> [w844 _ w851]
                  frame -1 {
                    n406 = global read "RIOGlobal.vi" "G_sel_disp"() -> (w850:u8)
                    n407 = Absolute Value(x=w844) -> (abs(x)=w845:dbl)
                    n408 = Not Equal?(x=w850, y=u8 7) -> (x != y?=w848:bool)
                    n409 = Select(t=0.0, s=w848, f=w845) -> (s? t:f=w846:dbl)
                  }
                  frame 0, Default {
                  }
                  frame 1 {
                    n410 = global read "RIOGlobal.vi" "G_sel_disp"() -> (w855:u8)
                    n411 = case shown="0, Default" w855 {
                      tunnel: [_ TRUE ("auto speed")] -> w854
                      frame 0, Default {
                      }
                      frame 1..3, 5 {
                      }
                    }
                    n412 = Select(t=w851, s=w854, f=0.0 ("t")) -> (s? t:f=w853:dbl)
                  }
                }
                n413 = global write "RIOGlobal.vi" "VS_Desire"(w840) -> ()
              }
              frame #1 {
                # "Throttle reverse Control"
                # "Throttle Control"
                n414 = call "rev_throttle.vi"() -> ()  [unwired: 11 in, 1 out]
                n415 = call "throttlecontroller2.vi"("Boolean"=TRUE) -> ()  [unwired: 11 in]
              }
            }
            n416 = Wait (ms)(milliseconds to wait=u32 5) -> ()  [unwired: 1 out]
          }
          n417 = while {
            tunnel: w673 -> [w688]
            stop <- FALSE stop-if-true
            n418 = flat-sequence {
              tunnel: w688 -> [w690]
              frame #0 {
                n419 = while {
                  tunnel: w690 -> [w697]
                  shift-right: [w699] -> _
                  shift-left: _ -> [w698]
                  shift-right: [w693] -> _
                  shift-left: i16 0 -> [w694]
                  stop <- w695 continue-if-true
                  n420 = global read "RIOGlobal.vi" "Auto"() -> (w700:bool)
                  n421 = case shown="True" w700 {
                    tunnel: [0.0 ("B Push percent x10") w736] -> w691
                    tunnel: w697 -> [_ w734]
                    tunnel: w694 -> [_ w733]
                    tunnel: [i16 0 ("y") w732] -> w693
                    tunnel: [FALSE w731] -> w692
                    frame False {
                    }
                    frame True {
                      n422 = global read "RIOGlobal.vi" "Run"() -> (w735:bool)
                      n423 = case shown="False" w735 {
                        tunnel: [w751 w767] -> w736
                        tunnel: w734 -> [_ w771]
                        tunnel: w733 -> [w749 _]
                        tunnel: [w740 i16 0 ("y")] -> w732
                        tunnel: [w739 FALSE] -> w731
                        frame False {
                          n424 = global read "RIOGlobal.vi" "Encoder 0"() -> (w742:dbl)
                          n425 = global read "RIOGlobal.vi" "Encoder"() -> (w744:dbl)
                          n426 = global read "RIOGlobal.vi" "VS_TCU"() -> (w753:dbl)
                          n427 = global read "RIOGlobal.vi" "Encoder percent"() -> (w737:dbl)
                          n428 = global read "RIOGlobal.vi" "Encoder 100"() -> (w743:dbl)
                          n429 = Subtract(x=w742, y=w743) -> (x-y=w745:dbl)
                          n430 = Divide(x=w744, y=w745) -> (x/y=w747:dbl)
                          n431 = Equal To 0?(x=w753) -> (x = 0?=w750:bool)
                          n432 = Multiply(x=100.0, y=w747) -> (x*y=w738:dbl)
                          n433 = case shown="True" w750 {
                            selector: w750 -> [_ w766]
                            tunnel: w749 -> [_ w764]
                            tunnel: [i16 0 ("y") w760] -> w740
                            tunnel: w738 -> [w758 _]
                            frame False {
                              n434 = Add(x=w758, y=5.0) -> (x+y=w756:dbl)
                              n435 = Max & Min(x=w756, y=100.0) -> (min(x,y)=w754:dbl)  [unwired: 1 out]
                              n436 = global write "RIOGlobal.vi" "Encoder percent"(w754) -> ()
                            }
                            frame True {
                              w761 = i16 40 ("y")
                              n437 = Boolean To (0,1)(Boolean=w766) -> (0, 1=w765:i16)
                              n438 = Add(x=w765, y=w764) -> (x+y=w762:i16)
                              n439 = Less?(x=w762, y=w761) -> (x < y?=w763:bool)
                              n440 = Select(t=w762, s=w763, f=w761) -> (s? t:f=w760:i16)
                            }
                          }
                          n441 = Increment(x=w737) -> (x+1=w741:dbl)
                          n442 = Equal?(x=w740, y=i16 40) -> (x = y?=w739:bool)
                          n443 = Select(t=w741, s=w739, f=100.0 ("B Push percent x10")) -> (s? t:f=w751:dbl)
                        }
                        frame True {
                          n444 = case shown="False" "auto brake" {
                            tunnel: [w774 w775] -> w767
                            tunnel: w771 -> [_ w783]
                            frame False {
                              n445 = call "lpf3.vi"("filter_gain"="brake filter", "In1"="Slide") -> ("Out1"=w774:dbl)  [unwired: 9 in]
                            }
                            frame True {
                              n446 = global read "RIOGlobal.vi" "VS_Desire"() -> (w779:dbl)
                              n447 = global read "RIOGlobal.vi" "VS_Desire"() -> (w778:dbl)
                              n448 = global read "RIOGlobal.vi" "VS_TCU"() -> (w782:dbl)
                              n449 = Subtract(x=w782, y=1.0 ("x-y")) -> (x-y=w780:dbl)
                              n450 = Subtract(x=w779, y=w780) -> (x-y=w784:dbl)
                              n451 = Equal To 0?(x=w778) -> (x = 0?=w777:bool)
                              n452 = Build Array(w784, w779) -> (w785:dbl[])
                              n453 = call-poly <vilib>:"FL Fuzzy Controller.vi"("input values"=w785, "fuzzy system in"=w783) -> ("output value"=w786:dbl)  [unwired: 5 in, 4 out]
                              n454 = Divide(x=w786, y=9.0) -> (x/y=w788:dbl)
                              n455 = Multiply(x=w788, y=12.0 ("brake")) -> (x*y=w776:dbl)
                              n456 = case shown="True" w777 {
                                tunnel: [w793 100.0 ("B Push percent x10")] -> w775
                                tunnel: w776 -> [w790 _]
                                frame False {
                                n457 = Max & Min(x=-50.0, y=w790) -> (max(x,y)=w792:dbl)  [unwired: 1 out]
                                n458 = Max & Min(x=w792, y=100.0) -> (min(x,y)=w793:dbl)  [unwired: 1 out]
                                }
                                frame True {
                                }
                              }
                            }
                          }
                        }
                      }
                    }
                  }
                  n459 = Wait (ms)(milliseconds to wait=u32 50) -> (millisecond timer value=w699:u32)
                  n460 = Subtract(x=w699, y=w698) -> (x-y=w696:u32)
                  n461 = global write "RIOGlobal.vi" "B ts"(w696) -> ()
                  n462 = flat-sequence {
                    tunnel: w692 -> [w714]
                    tunnel: w691 -> [w702]
                    frame #0 {
                      n463 = global read "RIOGlobal.vi" "G_sel_disp"() -> (w704:u8)
                      n464 = local read "auto brake"() -> (w712:bool)
                      n465 = global read "RIOGlobal.vi" "Encoder 0"() -> (w720:dbl)
                      n466 = global read "RIOGlobal.vi" "Encoder"() -> (w718:dbl)
                      n467 = global read "RIOGlobal.vi" "VS_TCU"() -> (w705:dbl)
                      n468 = global read "RIOGlobal.vi" "Encoder 100"() -> (w719:dbl)
                      n469 = Equal To 0?(x=w705) -> (x = 0?=w706:bool)
                      n470 = Equal To 0?(x=w704) -> (x = 0?=w707:bool)
                      n471 = Subtract(x=w720, y=w719) -> (x-y=w717:dbl)
                      n472 = And(x=w706, y=w707) -> (x .and. y?=w709:bool)
                      n473 = Divide(x=w718, y=w717) -> (x/y=w715:dbl)
                      n474 = Select(t=0.0, s=w709, f=w702) -> (s? t:f=w703:dbl)
                      "B Push percent x10" <- w703
                      n475 = Multiply(x=100.0, y=w715) -> (x*y=w713:dbl)
                      n476 = call "brakecontrol1.vi"("e-stop"=w714, "theta_encoder"=w713, "theta_des"=w703) -> ("Tm_ff[duty%]"=w711:dbl)  [unwired: 8 in]
                      n477 = case shown="False" w712 {
                        tunnel: w711 -> [w724 w727]
                        tunnel: [w721 w727] -> w710
                        frame False {
                          n478 = Absolute Value(x=w724) -> (abs(x)=w726:dbl)
                          n479 = Greater?(x=w726, y=5.0) -> (0:w722:bool)
                          n480 = Select(t=w724, s=w722, f=0.0) -> (s? t:f=w721:dbl)
                        }
                        frame True {
                        }
                      }
                      n481 = global write "RIOGlobal.vi" "B PWM"(w710) -> ()
                    }
                  }
                  n482 = global read "RIOGlobal.vi" "Auto"() -> (w695:bool)
                }
              }
              frame #1 {
                n483 = while {
                  shift-right: [w797] -> _
                  shift-left: TRUE -> [w798]
                  stop <- w811 stop-if-true
                  n484 = global read "RIOGlobal.vi" "Encoder 0"() -> (w805:dbl)
                  n485 = global read "RIOGlobal.vi" "Encoder"() -> (w807:dbl)
                  n486 = global read "RIOGlobal.vi" "Encoder 100"() -> (w806:dbl)
                  n487 = Subtract(x=w805, y=w806) -> (x-y=w808:dbl)
                  n488 = Divide(x=w807, y=w808) -> (x/y=w810:dbl)
                  n489 = Multiply(x=100.0, y=w810) -> (x*y=w804:dbl)
                  n490 = Greater Than 0?(x=w804) -> (x > 0?=w799:bool)
                  n491 = And(x=w799, y=w798) -> (x .and. y?=w797:bool)
                  n492 = Wait (ms)(milliseconds to wait=u32 5) -> ()  [unwired: 1 out]
                  n493 = Select(t=-20.0, s=w797, f=0.0) -> (s? t:f=w801:dbl)
                  n494 = global write "RIOGlobal.vi" "B PWM"(w801) -> ()
                  n495 = global read "RIOGlobal.vi" "Auto"() -> (w811:bool)
                }
              }
            }
          }
        }
      }
    }
  }
